vi "Configure Trigger (Rise Fall Time).vi"(0 "VISA resource name":refnum<visa-resource-name>, 1 "Trigger Slope (0: Rising)":u16(ring) items=["Rising", "Falling", "Either"], 5 "Trigger Source (0: Channel 1)":u16(ring) items=["Channel 1", "Channel 2", "Channel 3", "Channel 4"], 7 "High Threshold (0.8V)":dbl=0.8, 9 "Low Threshold (0.0V)":dbl, 11 "error in (no error)":errorcluster, 12 "Trigger Condition (0: Less Than)":u16(ring) items=["Less Than", "More Than", "Equal", "Not Equal"], 13 "Delta Time (4.0ns)":dbl=4e-09) -> (4 "VISA resource name out":refnum<visa-resource-name>, 15 "error out":errorcluster)   [LabVIEW 2016, in "Tektronix DPO MSO 2000 4000 Series.lvlib"]
doc: "Configures rise- and fall-time trigger settings."
uses:
  Tektronix DPO MSO 2000 4000 Series.lvlib
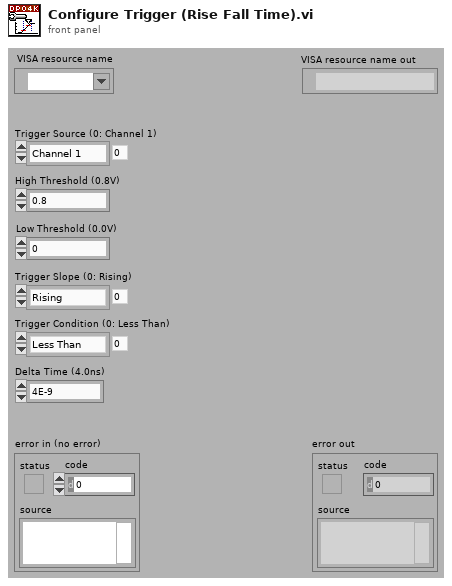
[diagram p1: front panel]
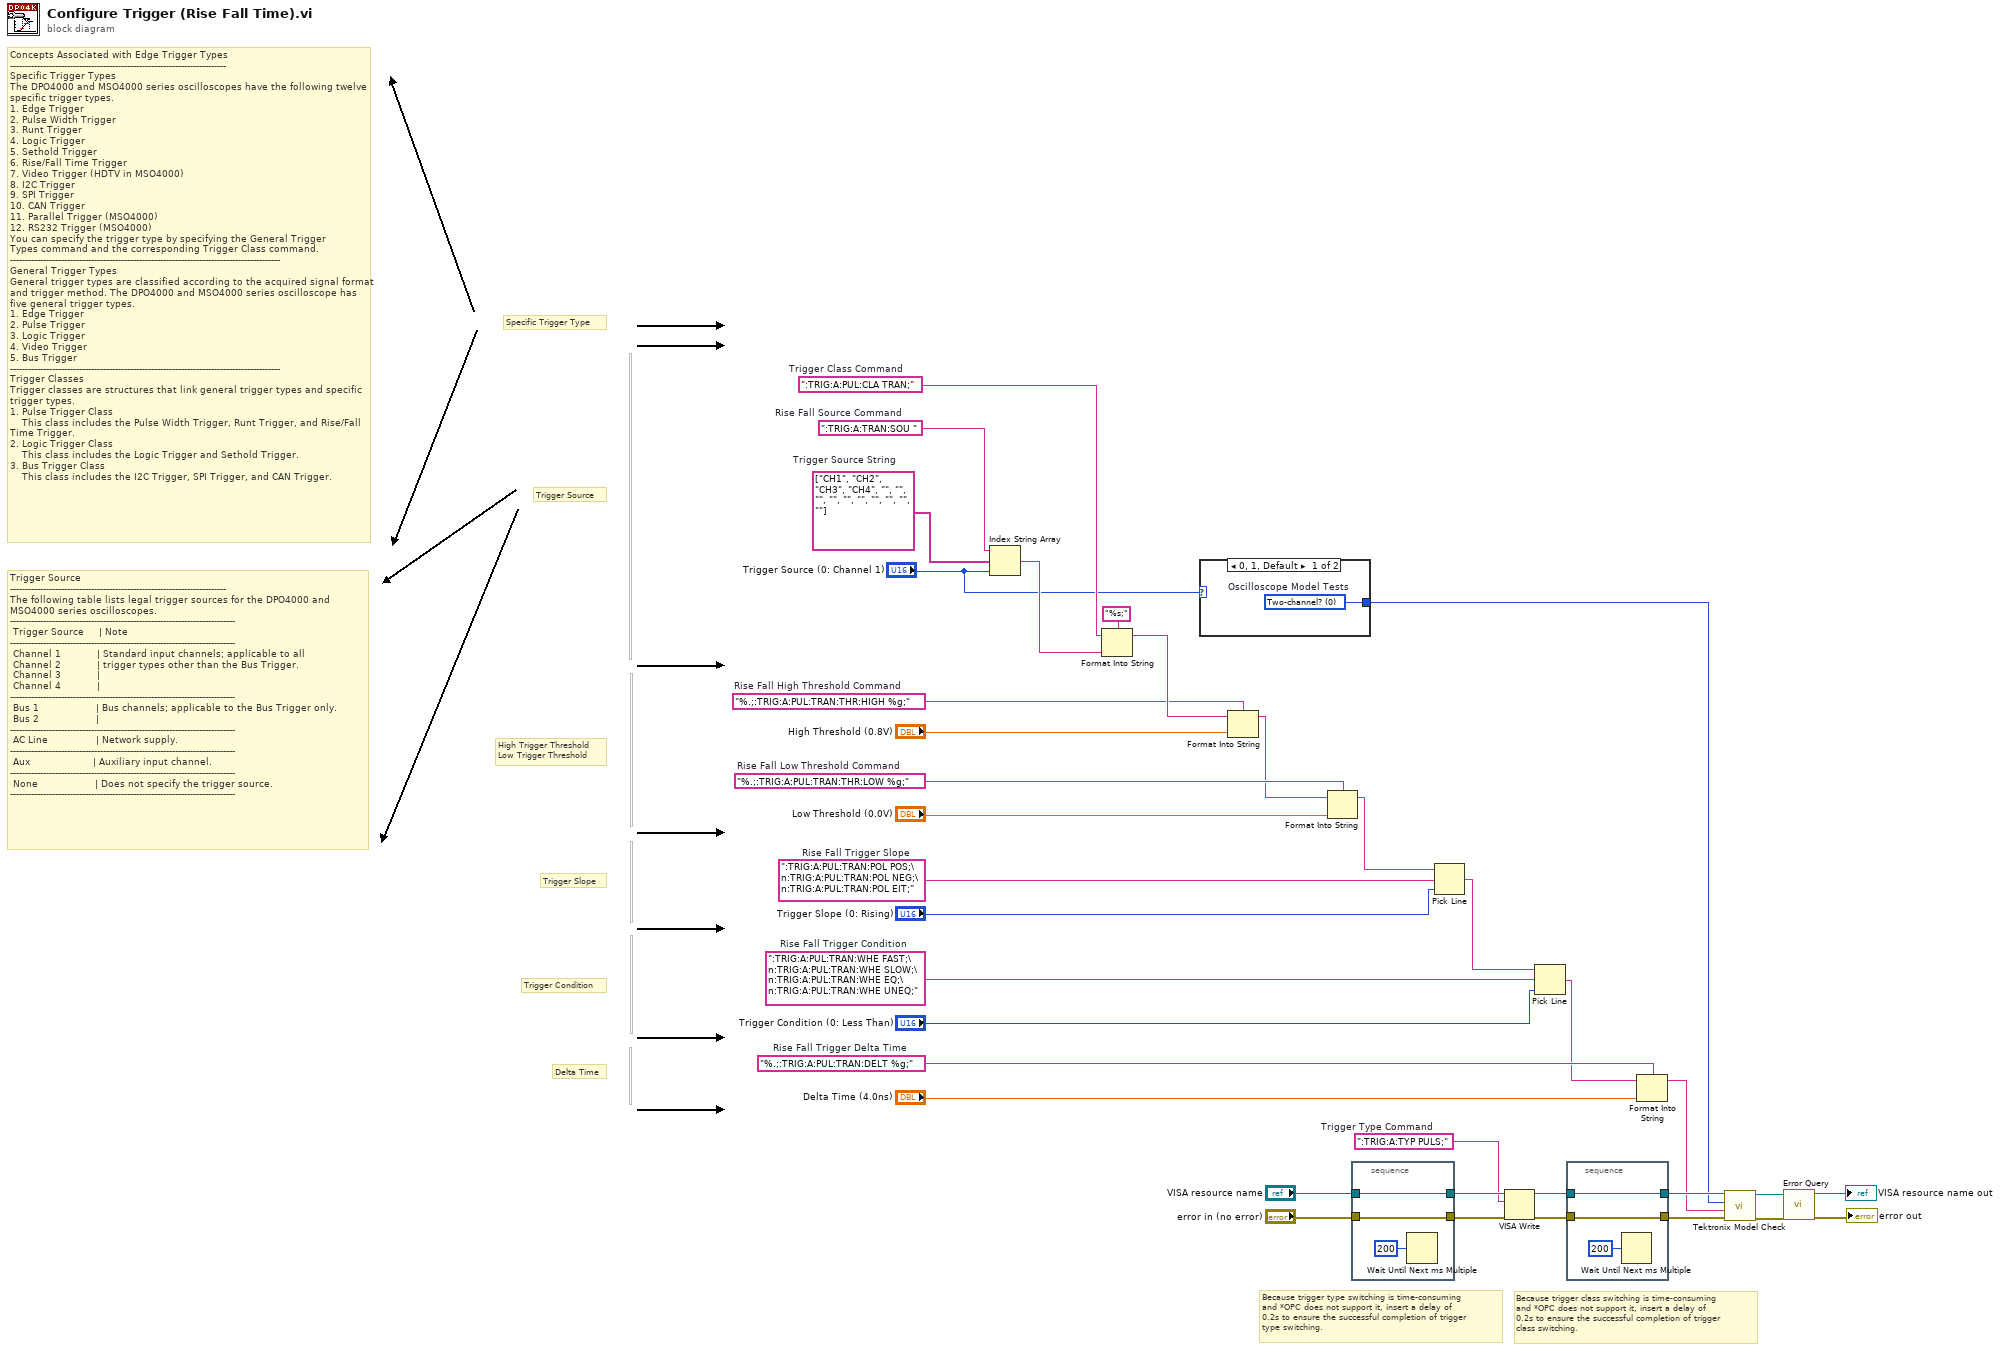
[diagram p0: block diagram]
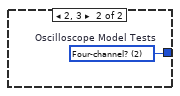
[diagram p2: hidden frame]
diagram:
  w10 = string[] ["CH1", "CH2", "CH3", "CH4", "", "", "", "", "", "", "", "", "", ""]  # Trigger Source String
  w14 = "%.;:TRIG:A:PUL:TRAN:DELT %g;"  # Rise Fall Trigger Delta Time
  w18 = ":TRIG:A:PUL:TRAN:WHE FAST;\n:TRIG:A:PUL:TRAN:WHE SLOW;\n:TRIG:A:PUL:TRAN:WHE EQ;\n:TRIG:A:PUL:TRAN:WHE UNEQ;"  # Rise Fall Trigger Condition
  w20 = ":TRIG:A:PUL:TRAN:POL POS;\n:TRIG:A:PUL:TRAN:POL NEG;\n:TRIG:A:PUL:TRAN:POL EIT;"  # Rise Fall Trigger Slope
  w23 = "%.;:TRIG:A:PUL:TRAN:THR:LOW %g;"  # Rise Fall Low Threshold Command
  w25 = "%.;:TRIG:A:PUL:TRAN:THR:HIGH %g;"  # Rise Fall High Threshold Command
  w31 = ":TRIG:A:TRAN:SOU "  # Rise Fall Source Command
  w34 = ":TRIG:A:TYP PULS;"  # Trigger Type Command
  w30 = ":TRIG:A:PUL:CLA TRAN;"  # Trigger Class Command
  # "Trigger Source\n------------------------------------------------------------------------\nThe following table lists legal trigger sources for the DPO4000 and MSO4000 series oscilloscopes.\n---------------------------------------------------------------------------\n Trigger Source     | Note                                                           \n---------------------------------------------------------------------------\n Channel 1            | Standard input channels; applicable to all      \n Channel 2            | trigger types other than the Bus Trigger.         \n Channel 3            |     \n Channel 4            |\n---------------------------------------------------------------------------\n Bus 1                   | Bus channels; applicable to the Bus Trigger only.\n Bus 2                   | \n---------------------------------------------------------------------------\n AC Line                | Network supply.\n---------------------------------------------------------------------------\n Aux                     | Auxiliary input channel.\n---------------------------------------------------------------------------\n None                   | Does not specify the trigger source.\n---------------------------------------------------------------------------"
  # "Concepts Associated with Edge Trigger Types\n------------------------------------------------------------------------\nSpecific Trigger Types\nThe DPO4000 and MSO4000 series oscilloscopes have the following twelve specific trigger types.\n1. Edge Trigger\n2. Pulse Width Trigger\n3. Runt Trigger\n4. Logic Trigger\n5. Sethold Trigger\n6. Rise/Fall Time Trigger\n7. Video Trigger (HDTV in MSO4000)\n8. I2C Trigger\n9. SPI Trigger\n10. CAN Trigger\n11. Parallel Trigger (MSO4000)\n12. RS232 Trigger (MSO4000)\nYou can specify the trigger type by specifying the General Trigger \nTypes command and the corresponding Trigger Class command.\n------------------------------------------------------------------------------------------\nGeneral Trigger Types \nGeneral trigger types are classified according to the acquired signal format and trigger method. The DPO4000 and MSO4000 series oscilloscope has five general trigger types.\n1. Edge Trigger\n2. Pulse Trigger\n3. Logic Trigger\n4. Video Trigger\n5. Bus Trigger\n------------------------------------------------------------------------------------------\nTrigger Classes\nTrigger classes are structures that link general trigger types and specific trigger types.\n1. Pulse Trigger Class\n    This class includes the Pulse Width Trigger, Runt Trigger, and Rise/Fall Time Trigger.\n2. Logic Trigger Class\n    This class includes the Logic Trigger and Sethold Trigger.\n3. Bus Trigger Class\n    This class includes the I2C Trigger, SPI Trigger, and CAN Trigger."
  # "Because trigger class switching is time-consuming\nand *OPC does not support it, insert a delay of\n0.2s to ensure the successful completion of trigger\nclass switching."
  # "Because trigger type switching is time-consuming\nand *OPC does not support it, insert a delay of\n0.2s to ensure the successful completion of trigger\ntype switching."
  # "Delta Time"
  # "Trigger Condition"
  # "Trigger Slope"
  # "High Trigger Threshold\nLow Trigger Threshold"
  # "Trigger Source"
  # "Specific Trigger Type"
  n1 = Index String Array(1:"Trigger Source (0: Channel 1)", 2:w10, 3:w31) -> (0:w29:string)
  n2 = Format Into String(format string="%s;", initial string=w30, w29) -> (resulting string=w27:string)  [unwired: 1 in, 1 out]
  n3 = case shown="0, 1, Default" "Trigger Source (0: Channel 1)" {
    tunnel: [w37 w38] -> w1
    frame 0, 1, Default {
      w37 = u16 0 items=["Two-channel?", "Digital Model?", "Four-channel?", "RF Model?"]  # Oscilloscope Model Tests
    }
    frame 2, 3 {
      w38 = u16 2 items=["Two-channel?", "Digital Model?", "Four-channel?", "RF Model?"]  # Oscilloscope Model Tests
    }
  }
  n4 = Format Into String(format string=w25, initial string=w27, "High Threshold (0.8V)") -> (resulting string=w22:string)  [unwired: 1 in, 1 out]
  n5 = Format Into String(format string=w23, initial string=w22, "Low Threshold (0.0V)") -> (resulting string=w21:string)  [unwired: 1 in, 1 out]
  n6 = stacked-sequence {
    tunnel: "VISA resource name" -> [w40]
    tunnel: [w40] -> w36
    tunnel: "error in (no error)" -> [w39]
    tunnel: [w39] -> w35
    frame #0 {
      n7 = Wait Until Next ms Multiple(millisecond multiple=u32 200) -> ()  [unwired: 1 out]
    }
  }
  n8 = Pick Line(string ("")=w21, multi-line string=w20, line index="Trigger Slope (0: Rising)") -> (output string=w16:string)
  n9 = VISA Write(VISA resource name=w36, write buffer=w34, error in (no error)=w35) -> (VISA resource name out=w33:refnum<visa-resource-name>, error out=w32:errorcluster)  [unwired: 1 out]
  n10 = Pick Line(string ("")=w16, multi-line string=w18, line index="Trigger Condition (0: Less Than)") -> (output string=w13:string)
  n11 = stacked-sequence {
    tunnel: w33 -> [w43]
    tunnel: [w43] -> w7
    tunnel: w32 -> [w42]
    tunnel: [w42] -> w6
    frame #0 {
      n12 = Wait Until Next ms Multiple(millisecond multiple=u32 200) -> ()  [unwired: 1 out]
    }
  }
  n13 = Format Into String(format string=w14, initial string=w13, "Delta Time (4.0ns)") -> (resulting string=w5:string)  [unwired: 1 in, 1 out]
  n14 = call "Tektronix Model Check.vi"("error in (no error)"=w6, "Command String"=w5, "Oscilloscope Model Tests (3: RF Model?)"=w1, "VISA resource name"=w7) -> ("error out"=w3:errorcluster, "VISA resource name out"=w4:refnum<visa-resource-name>)  [unwired: 6 in]
  n15 = call "Error Query.vi"("error in (no error)"=w3, "VISA resource name"=w4) -> ("error out"=→"error out":errorcluster, "VISA resource name out"=→"VISA resource name out":refnum<visa-resource-name>)  [unwired: 6 in, 2 out]
